vi "ConfigurePiePlot.vi"(0 "reference in":refnum<class "HTMLPlot.lvclass">, 5 "error in (no error)":errorcluster) -> (14 "reference out":refnum<class "HTMLPlot.lvclass">, 16 "fullHTML":string, 19 "error out":errorcluster)   [LabVIEW 2019, in "HTMLPlot.lvclass"]
uses:
  HTMLPlot.lvclass
panel:
  out "plotOptions":string
  out "plotData":string
  out "plotType":string
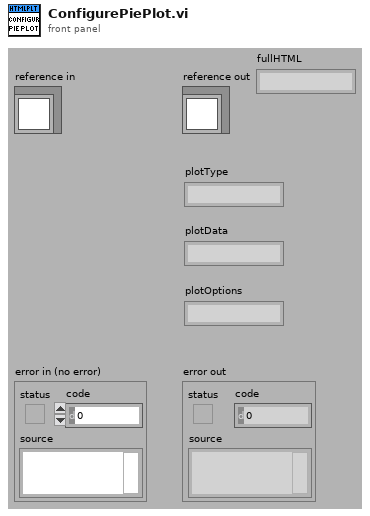
[diagram p1: front panel]
types:
  T1 = typedef "HTMLPlot.lvclass/ObjectAttributes.ctl" = cluster{"Attribute1":dbl, "GraphContainer":refnum<k7>, "ChartScriptFile":string, "UtilScriptFile(demoData)":string, "BaseHTML":string, "GenericProperties":cluster{"PlotType":T2, "PlotTitle":string, "XLabel":string, "YLabel":string, "ShowToolTip":bool}, "LegendProperties":cluster{"Show":bool, "Position":T3}, "BarPlot":cluster{"Dataset":dbl[][], "DatasetLabels":string[], "XLabels":string[], "PlotColours":u32[], "Stacked":bool}, "PiePlot":cluster{"Dataset":dbl[][], "DatasetLabels":string[], "PlotColours":u32[], "DoughnutStyle":bool, "PlotLabels":string[]}, "connection ID":refnum<k5>, "PortID":u64}
  T2 = typedef "HTMLPlot.lvclass/PlotType.ctl" = enum16{"bar", "line", "pie"}
  T3 = typedef "HTMLPlot.lvclass/LegendPosition.ctl" = enum16{"top", "right", "left", "bottom"}
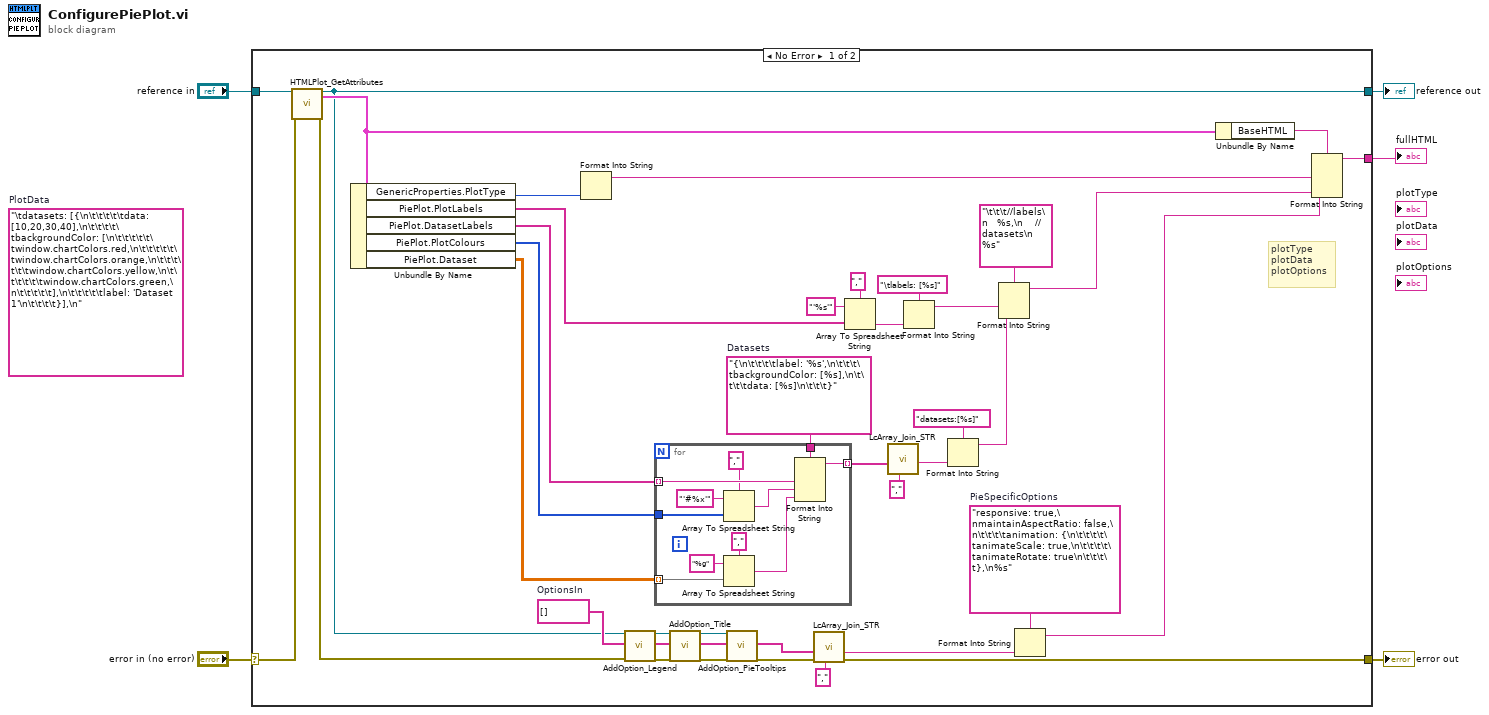
[diagram p0: block diagram]
diagram:
  (unwired) "\tdatasets: [{\n\t\t\t\t\tdata: [10,20,30,40],\n\t\t\t\t\tbackgroundColor: [\n\t\t\t\t\t\twindow.chartColors.red,\n\t\t\t\t\t\twindow.chartColors.orange,\n\t\t\t\t\t\twindow.chartColors.yellow,\n\t\t\t\t\t\twindow.chartColors.green,\n\t\t\t\t\t],\n\t\t\t\t\tlabel: 'Dataset 1'\n\t\t\t\t}],\n"  # PlotData
  n1 = case shown="No Error" "error in (no error)" {
    selector: "error in (no error)" -> [w45 w58]
    tunnel: [w16 w58] -> w4
    tunnel: [w20 w57] -> w2
    tunnel: "reference in" -> [w44 w57]
    tunnel: [w15 _] -> w1
    frame No Error {
      w9 = "responsive: true,\nmaintainAspectRatio: false,\n\t\t\t\tanimation: {\n\t\t\t\t\tanimateScale: true,\n\t\t\t\t\tanimateRotate: true\n\t\t\t\t},\n%s"  # PieSpecificOptions
      w24 = "{\n\t\t\t\tlabel: '%s',\n\t\t\t\tbackgroundColor: [%s],\n\t\t\t\tdata: [%s]\n\t\t\t}"  # Datasets
      w30 = string[] []  # OptionsIn
      # "plotType\nplotData\nplotOptions"
      n2 = call "HTMLPlot_GetAttributes.vi"("reference in"=w44, "error in (no error)"=w45) -> ("reference out"=w20:refnum<class "HTMLPlot.lvclass">, "Data"=w23:T1, "error out"=w17:errorcluster)  [unwired: 14 in, 1 out]
      n3 = Unbundle By Name(w23) -> ("GenericProperties.PlotType"=w22:T2, "PiePlot.PlotLabels"=w6:string[], "PiePlot.DatasetLabels"=w36:string[], "PiePlot.PlotColours"=w37:u32[], "PiePlot.Dataset"=w18:dbl[][])
      n4 = Format Into String(w22) -> (resulting string=w21:string)  [unwired: 3 in, 1 out]
      n5 = call "AddOption_Legend.vi"("reference in"=w20, "OptionsIn"=w30, "error in (no error)"=w17) -> ("reference out"=w29:refnum<class "HTMLPlot.lvclass">, "OptionsOut"=w28:string[], "error out"=w27:errorcluster)  [unwired: 14 in]
      n6 = for {
        tunnel: w18 -> [w54] mode=indexing
        tunnel: w37 -> [w47]
        tunnel: w36 -> [w53] mode=indexing
        tunnel: [w51] -> w34 mode=indexing
        tunnel: w24 -> [w50]
        n7 = Array To Spreadsheet String(delimiter (Tab)=",", array=w47, 3:"'#%x'" ("format string")) -> (spreadsheet string=w46:string)
        n8 = Array To Spreadsheet String(delimiter (Tab)=",", array=w54, 3:"%g" ("format string")) -> (spreadsheet string=w52:string)
        n9 = Format Into String(format string=w50, w53, w46, w52) -> (resulting string=w51:string)  [unwired: 2 in, 1 out]
      }
      n10 = call "AddOption_Title.vi"("reference in"=w29, "OptionsIn"=w28, "error in (no error)"=w27) -> ("reference out"=w10:refnum<class "HTMLPlot.lvclass">, "OptionsOut"=w11:string[], "error out"=w12:errorcluster)  [unwired: 14 in]
      n11 = call "AddOption_PieTooltips.vi"("reference in"=w10, "OptionsIn"=w11, "error in (no error)"=w12) -> ("OptionsOut"=w14:string[], "error out"=w13:errorcluster)  [unwired: 14 in, 1 out]
      n12 = call "LcArray_Join_STR.vi"("separator"=",", "error in (no error)"=w13, "Array"=w14) -> ("error out"=w16:errorcluster, "joined string"=w8:string)  [unwired: 7 in]
      n13 = Array To Spreadsheet String(delimiter (Tab)=",", array=w6, 3:"'%s'" ("format string")) -> (spreadsheet string=w38:string)
      n14 = call "LcArray_Join_STR.vi"("separator"=",", "Array"=w34) -> ("joined string"=w33:string)  [unwired: 8 in, 1 out]
      n15 = Format Into String(format string="\tlabels: [%s]", w38) -> (resulting string=w41:string)  [unwired: 2 in, 1 out]
      n16 = Format Into String(format string="datasets:[%s]", w33) -> (resulting string=w31:string)  [unwired: 2 in, 1 out]
      n17 = Format Into String(format string="\t\t\t//labels\n   %s,\n    //datasets\n   %s", w41, w31) -> (resulting string=w19:string)  [unwired: 2 in, 1 out]
      n18 = Format Into String(format string=w9, w8) -> (resulting string=w7:string)  [unwired: 2 in, 1 out]
      n19 = Unbundle By Name(w23) -> ("BaseHTML"=w43:string)
      n20 = Format Into String(format string=w43, w21, w19, w7) -> (resulting string=w15:string)  [unwired: 2 in, 1 out]
    }
    frame Error {
    }
  }
  "error out" <- w4
  "reference out" <- w2
  "fullHTML" <- w1
